vi "Check for Disabled Devices before Compile.vi"(8 "error in (no error)":errorcluster, 11 "Ballard ARINC 429 ref":T1 format="%.0x") -> (0 "error out":errorcluster, 2 "Custom Device is Disabled":bool, 3 "Ballard ARINC 429 ref":T1 format="%.0x")   [LabVIEW 2020, in "Ballard ARINC 429 System Explorer.lvlib" / "Implementation.lvlib"]
uses:
  Implementation.lvlib
  <vilib>/NI VeriStand/Custom Device API/Custom Device Item Ref.ctl
  Scripting/Ballard/Constants.vi
  <vilib>/NI VeriStand/Custom Device API/Custom Device API.lvlib
  Scripting/Ballard/Ballard ARINC 429 Scripting.lvlib
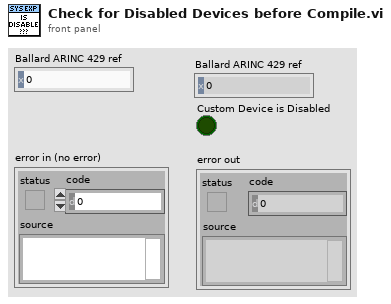
[diagram p1: front panel]
types:
  T1 = typedef "Custom Device API.lvlib/Custom Device Item Ref.ctl" = u64
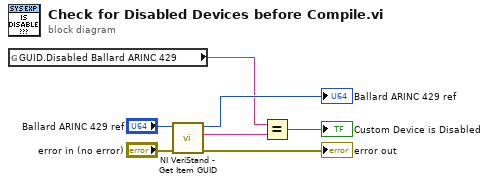
[diagram p0: block diagram]
diagram:
  n1 = global read "Constants.vi" "GUID.Disabled Ballard ARINC 429"() -> (w3:string)
  n2 = call <vilib>:"NI VeriStand - Get Item GUID.vi"("error in (no error)"="error in (no error)", "Item Ref in"="Ballard ARINC 429 ref") -> ("error out"=→"error out":errorcluster, "GUID"=w2:string, "Item Ref out"=→"Ballard ARINC 429 ref":T1)  [unwired: 7 in]
  n3 = Equal?(x=w3, y=w2) -> (x = y?=→"Custom Device is Disabled":bool)
